vi "Rotation2d_GetAngleCosSin.vi"(11 "in ROTATION":T1={"VALUE"=0.0, "COS"=1.0, "SIN"=0.0} {"SIN" format="%13.4f"; "COS" format="%13.4f"; "VALUE" format="%13.4f"}) -> (1 "Cosine":dbl, 2 "Sine":dbl, 3 "Angle":dbl)   [LabVIEW 2019, in "Trajectory_Library.lvlib"]
doc: "Returns the angle, sine, and cosine of the rotation.\n\nParameters:\n - in ROTATION - This ROTATION data structure\n\nReturns:\n - Angle - The angle of the ROTATION (radians)\n - Cosine of the ROTATAION\n - Sine of the ROTATAION"
uses:
  Trajectory_Library.lvlib
  ROTATION2D.ctl
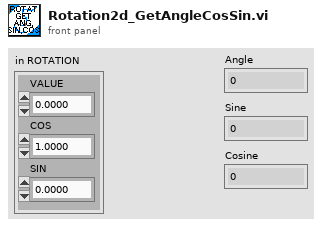
[diagram p1: front panel]
types:
  T1 = typedef "Trajectory_Library.lvlib/ROTATION2D.ctl" = cluster{"VALUE":dbl, "COS":dbl, "SIN":dbl}
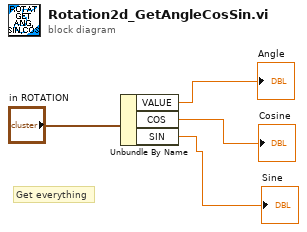
[diagram p0: block diagram]
diagram:
  # "Get everything"
  n1 = Unbundle By Name("in ROTATION") -> ("VALUE"=→"Angle":dbl, "COS"=→"Cosine":dbl, "SIN"=→"Sine":dbl)
